vi "Initialize.vi"(6 "EF ID":string, 7 "Base ID":string, 8 "error in (no error)":errorcluster, 10 "Motor IDs":string[](array[string]), 11 "Robot ID":string) -> (0 "error out":errorcluster, 3 "Simu Delta Robot":refnum<class "Simu Delta Robot.lvclass">)   [LabVIEW 2013, in "Simu Delta Robot.lvclass"]
uses:
  Simu Delta Robot.lvclass
  Simu Delta Robot.lvclass/Simu Delta Robot.ctl
  <vilib>/robotics/Simulator/Interface/Simulator References/Get Robot Component Reference.vi
  <instrlib>/Hitec HS400 Series/HAIOL/Hitec HS400 Series.lvclass
  <instrlib>/Hitec HS400 Series/HAIOL/Simulator/Hitec HS400 Series Simulator.lvclass
  <vilib>/robotics/Simulator/NI_Robotics_Simulator.lvlib
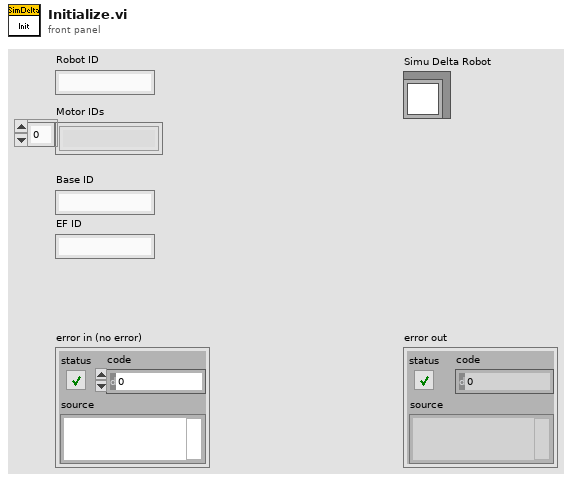
[diagram p1: front panel]
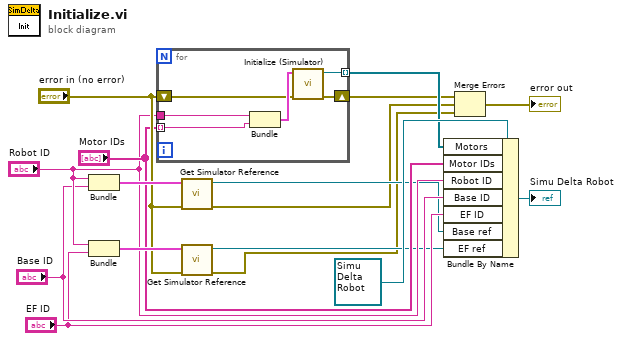
[diagram p0: block diagram]
diagram:
  n1 = Bundle("Robot ID"="Robot ID", "Base ID"="Base ID") -> (w15:cluster{"Robot ID":string, "Base ID":string})  [unwired: 1 in]
  n2 = Bundle("Robot ID"="Robot ID", "EF ID"="EF ID") -> (w14:cluster{"Robot ID":string, "EF ID":string})  [unwired: 1 in]
  n3 = for {
    tunnel: "Robot ID" -> [w22]
    tunnel: "Motor IDs" -> [w21] mode=indexing
    shift-right: [w18] -> w4
    shift-left: "error in (no error)" -> [w19]
    tunnel: [w17] -> w12 mode=indexing
    n4 = Bundle("Robot ID"=w22, "Motor ID"=w21) -> (w20:cluster{"Robot ID":string, "Motor ID":string})  [unwired: 1 in]
    n5 = call <instrlib>:"Initialize (Simulator).vi"("error in (no error)"=w19, "Device ID"=w20) -> ("error out"=w18:errorcluster, "Hitec HS400 Series out"=w17:refnum<class "Hitec HS400 Series.lvclass">)  [unwired: 8 in]
  }
  n6 = call-poly <vilib>:"Get Simulator Reference.vi"("error in (no error)"="error in (no error)", "robot component ID"=w15) -> ("error out"=w3:errorcluster, "component ref"=w7:refnum<k20>)  [unwired: 8 in]
  n7 = call-poly <vilib>:"Get Simulator Reference.vi"("error in (no error)"="error in (no error)", "robot component ID"=w14) -> ("error out"=w2:errorcluster, "component ref"=w6:refnum<k20>)  [unwired: 8 in]
  n8 = Bundle By Name(cluster=refnum<class "Simu Delta Robot.lvclass"> refnum ("Simu Delta Robot.lvclass"), "Motors"=w12, "Motor IDs"="Motor IDs", "Robot ID"="Robot ID", "Base ID"="Base ID", "EF ID"="EF ID", "Base ref"=w7, "EF ref"=w6) -> (→"Simu Delta Robot":refnum<class "Simu Delta Robot.lvclass">)
  n9 = Merge Errors(w4, w3, w2) -> (→"error out":errorcluster)
